vi "Recursive find Children.vi"(7 "Parent Class Path":path, 8 "error in (no error)":errorcluster, 10 "Classes":refnum<vi>[](array[refnum]), 11 "Class Map In":map{string, path}(c390)) -> (0 "error out":errorcluster, 3 "Class Map":map{string, path}(c390))   [LabVIEW 2020, in "New Class Dialog.lvclass"]
uses:
  New Class Dialog.lvclass
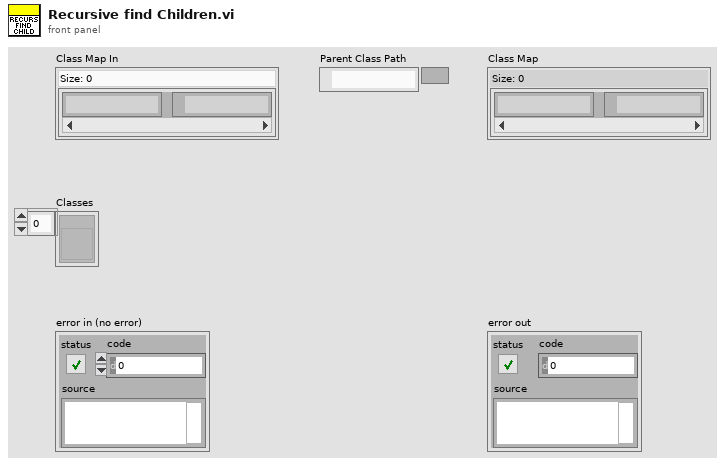
[diagram p1: front panel]
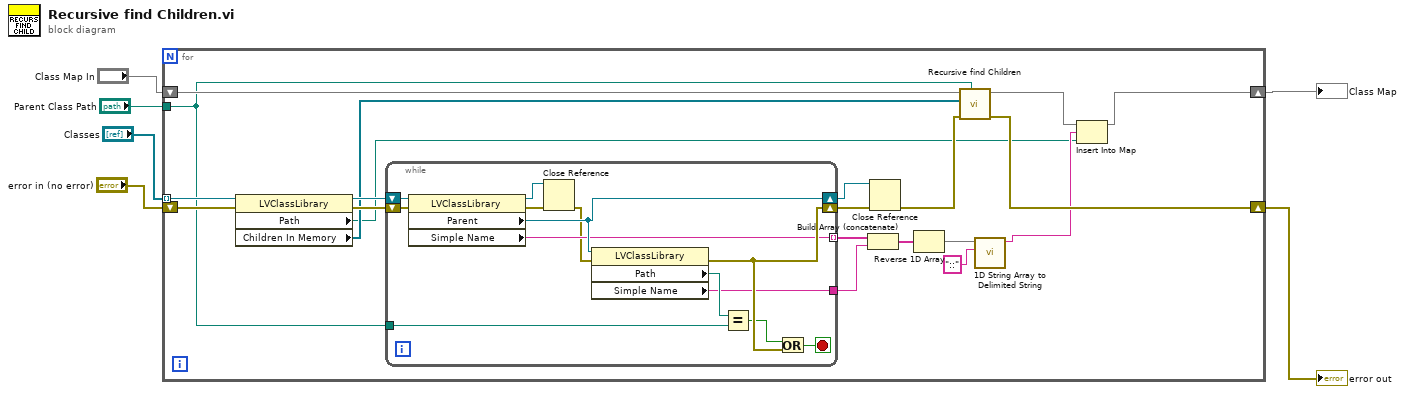
[diagram p0: block diagram]
diagram:
  n1 = for {
    tunnel: "Classes" -> [w20] mode=indexing
    shift-right: [w13] -> w6
    shift-left: "error in (no error)" -> [w17]
    tunnel: "Parent Class Path" -> [w7]
    shift-right: [w10] -> w2
    shift-left: "Class Map In" -> [w12]
    n2 = property class="LVClassLibrary"(reference=w20, error in=w17) -> (reference out=w19:refnum<vi>, error out=w18:errorcluster, "Path"=w8:path, "Children In Memory"=w15:refnum<vi>[])
    n3 = while {
      tunnel: w7 -> [w37]
      shift-right: [w34] -> w26
      shift-left: w18 -> [w36]
      shift-right: [w32] -> w16
      shift-left: w19 -> [w39]
      tunnel: [w31] -> w24 mode=indexing
      tunnel: [w30] -> w25
      stop <- w35 stop-if-true
      n4 = property class="LVClassLibrary"(reference=w39, error in=w36) -> (reference out=w27:refnum<vi>, error out=w33:errorcluster, "Parent"=w32:refnum<vi>, "Simple Name"=w31:string)
      n5 = Close Reference(reference=w27, error in (no error)=w33) -> (error out=w28:errorcluster)
      n6 = property class="LVClassLibrary"(reference=w32, error in=w28) -> (error out=w34:errorcluster, "Path"=w38:path, "Simple Name"=w30:string)  [unwired: 1 out]
      n7 = Equal?(x=w38, y=w37) -> (x = y?=w29:bool)
      n8 = Or(x=w29, y=w34) -> (x .or. y?=w35:bool)
    }
    n9 = Build Array (concatenate)(w24, w25) -> (w23:string[])
    n10 = Close Reference(reference=w16, error in (no error)=w26) -> (error out=w14:errorcluster)
    n11 = Reverse 1D Array(array=w23) -> (reversed array=w22:string[])
    n12 = call "Recursive find Children.vi"("Parent Class Path"=w7, "error in (no error)"=w14, "Classes"=w15, "Class Map In"=w12) -> ("error out"=w13:errorcluster, "Class Map"=w11:map{string, path})  [unwired: 6 in]
    n13 = call <vilib>:"1D String Array to Delimited String.vi"("delimiter"="::", "string array"=w22) -> ("delimited string"=w9:string)  [unwired: 9 in]
    n14 = Insert Into Map(map in=w11, key=w9, value=w8) -> (map out=w10:map{string, path})  [unwired: 2 out]
  }
  "error out" <- w6
  "Class Map" <- w2
